vi "XIPIN_Image_Statistics_2_0.vi"   [LabVIEW 2017]
doc: "The Xilinx Image Statistics LogiCORE collects statistical information for each video frame. This core generates a set of statistics for color histograms, mean and variance values, edge, and frequency content for 16 user defined zones on a per frame basis. The statistical information collected can be used in control loops for Auto-Focus, Auto-White Balance and Auto-Exposure applications.\n------------------------------------\n<b>Need License</b> : Yes"
uses:
  <vilib>/rvi/XilinxIP/XIPIN_XNode/niFpgaXIPIN.xnode
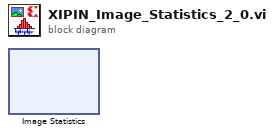
[diagram p0: block diagram]
diagram:
  n1 = xnode ("Image Statistics")() -> ()
